vi "E2 Data Logger.vi"(7 "refnum in":refnum<file>) -> (3 "refnum out":refnum<file>)   [LabVIEW 2014]
uses:
  <vilib>/Rock Robotics/WPI/DriverStation/WPI_DriverStationRobotMode2.ctl
  Robot Global Data.vi
  Moose Code/Auto_Conf.vi
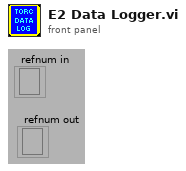
[diagram p1: front panel]
types:
  T1 = typedef "WPI_DriverStationRobotMode2.ctl" = enum16{"Autonomous Disabled", "Autonomous Enabled", "Teleop Disabled", "Teleop Enabled", "Disconnected", "Finish", "Test Disabled", "Test Enabled", "Emergency Stopped"}
  T2 = enum16{"ResetForward", "ResetBack", "PIDControl", "ManualControl", "ZeroEncoderAndTarget", "AutoStack"}
  T3 = enum16{"Disabled", "Initialize", "CalcNewTarget", "Moving", "OpenArm", "CloseArm", "Reset"}
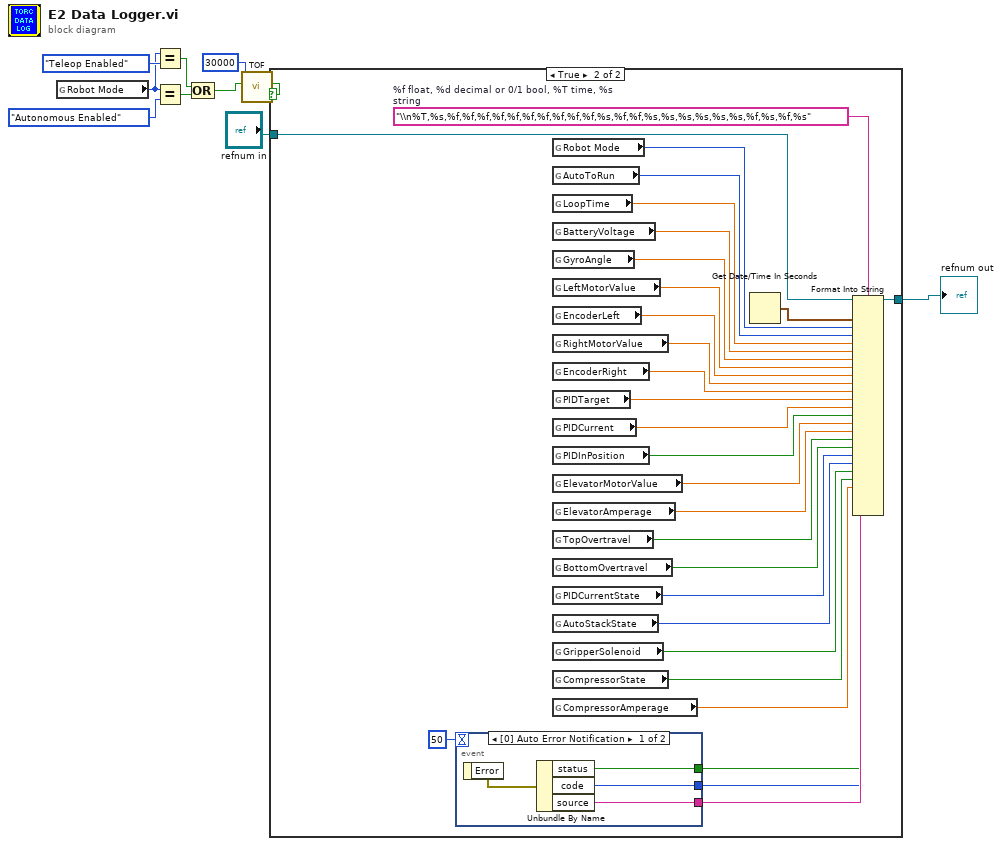
[diagram p0: block diagram]
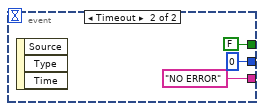
[diagram p3: hidden frame]
diagram:
  n1 = global read "Robot Global Data.vi" "Robot Mode"() -> (w4:T1)
  n2 = Equal?(x=w4, y=WPI_DriverStationRobotMode2."Teleop Enabled") -> (x = y?=w6:bool)
  n3 = Equal?(x=w4, y=WPI_DriverStationRobotMode2."Autonomous Enabled") -> (x = y?=w5:bool)
  n4 = Compound Arithmetic op=OR(w6, w5) -> (w3:bool)
  n5 = call "TOF.vi"("Delay (ms)"=u32 30000, "Input"=w3) -> ("Output"=w2:bool)  [unwired: 9 in]
  n6 = case shown="True" w2 {
    tunnel: [w11 w40] -> w10
    tunnel: "refnum in" -> [w11 w16]
    frame False {
    }
    frame True {
      w37 = "\\n%T,%s,%f,%f,%f,%f,%f,%f,%f,%f,%f,%f,%s,%f,%f,%s,%s,%s,%s,%s,%s,%f,%s,%f,%s"  # %f float, %d decimal or 0/1 bool, %T time, %s string
      n7 = event shown="[0] Auto Error Notification" {
        selector: _ -> [_ _]
        dyn-events: _ -> [_ _]
        timeout: 50 -> [_ _]
        tunnel: [w43 "NO ERROR" ("source")] -> w15
        tunnel: [w42 0 ("code")] -> w14
        tunnel: [w41 FALSE ("status")] -> w12
        event Auto Error Notification {
          n8 = event-data() -> ("Error"=w44:errorcluster)  [unwired: 1 in]
          n9 = Unbundle By Name(w44) -> ("status"=w41:bool, "code"=w42:i32, "source"=w43:string)
        }
        event Timeout {
          n10 = event-data() -> ()  [unwired: 1 in, 3 out]
        }
      }
      n11 = global read "Robot Global Data.vi" "Robot Mode"() -> (w38:T1)
      n12 = global read "Auto_Conf.vi" "AutoToRun"() -> (w36:u8)
      n13 = global read "Robot Global Data.vi" "LoopTime"() -> (w35:dbl)
      n14 = global read "Robot Global Data.vi" "BatteryVoltage"() -> (w34:dbl)
      n15 = global read "Robot Global Data.vi" "GyroAngle"() -> (w33:dbl)
      n16 = global read "Robot Global Data.vi" "LeftMotorValue"() -> (w32:dbl)
      n17 = global read "Robot Global Data.vi" "EncoderLeft"() -> (w31:dbl)
      n18 = global read "Robot Global Data.vi" "RightMotorValue"() -> (w30:dbl)
      n19 = global read "Robot Global Data.vi" "EncoderRight"() -> (w29:dbl)
      n20 = global read "Robot Global Data.vi" "PIDTarget"() -> (w28:dbl)
      n21 = global read "Robot Global Data.vi" "PIDCurrent"() -> (w27:dbl)
      n22 = global read "Robot Global Data.vi" "PIDInPosition"() -> (w26:bool)
      n23 = global read "Robot Global Data.vi" "ElevatorMotorValue"() -> (w25:dbl)
      n24 = global read "Robot Global Data.vi" "ElevatorAmperage"() -> (w24:dbl)
      n25 = global read "Robot Global Data.vi" "TopOvertravel"() -> (w23:bool)
      n26 = global read "Robot Global Data.vi" "BottomOvertravel"() -> (w22:bool)
      n27 = global read "Robot Global Data.vi" "PIDCurrentState"() -> (w21:T2)
      n28 = global read "Robot Global Data.vi" "AutoStackState"() -> (w20:T3)
      n29 = global read "Robot Global Data.vi" "GripperSolenoid"() -> (w19:bool)
      n30 = global read "Robot Global Data.vi" "CompressorState"() -> (w18:bool)
      n31 = global read "Robot Global Data.vi" "CompressorAmperage"() -> (w17:dbl)
      n32 = Get Date/Time In Seconds() -> (seconds since 1Jan1904=w39:timestamp)
      n33 = Format Into String(format string=w37, initial string=w16, w39, w38, w36, w35, w34, w33, w32, w31, w30, w29, w28, w27, w26, w25, w24, w23, w22, w21, w20, w19, w18, w17, w12, w14, w15) -> (resulting string=w40:refnum<file>)  [unwired: 1 in, 1 out]
    }
  }
  "refnum out" <- w10
